vi "LabViewV1.0.0.vi"() -> ()   [LabVIEW 2020]
uses:
  <vilib>/DAQmx/read.llb/DAQmx Read (Analog 2D DBL NChan NSamp).vi
  <vilib>/Analysis/baseanly.llb/Mean (DBL).vi
  <vilib>/DAQmx/miscellaneous.llb/DAQmx Fill In Error Info.vi
  <vilib>/Analysis/NI_AALBase.lvlib
  <resource>/objmgr/daqmx.rc
panel:
  out "Numeric 2":i32
  out "Numeric":i32
  out "index of Module 3":i32
  out "index of Module 2":i32
  out "double precision float":dbl
  out "Time Stamp":timestamp=timestamp(-21600 s since 1904-01-01)
  out "subarray 2":string[](array[string])
  out "index of Module 1":i32
  out "subarray":string[](array[string])
  in  "Counter":dbl
  out ".not. (x .or. y)?":bool
  out "index of element":i32
  out "element":dbl
  out "?":timestamp
  out "Channels":refnum<k21>[](array[refnum])
  out "size(s)":i32
  out "NumDevices":u32
  out "x/y":dbl
  in  "?":T1(tab)
  out "Sampling Status":bool
  in  "Sampling Time":u32=5
  in  "Read Time (s)":u32=60
  in  "Channel List":string(combo)="Temperature"
  out "Read Count Daily":string="0" caption="Timestamp"
  out "Countdown to Read":string="0\n 6:17:48 PM" caption="Timestamp"
  out "?":string="Timestamp"
  out "?":string="File Location"
  out "Timestamp":string="7/26/2020\n 6:17:48 PM"
  in  "Start":bool
  in  "Next Button":bool
  in  "Stop Button 2":bool
  out "Graph Running":bool
  in  "Resolution":u8=10 min=10
  in  "Stop Button":bool
  in  "Play Button":bool
  out "Module 3":bool
  out "Module 2":bool
  out "Module 1":bool
  out "3":bool
  out "2":bool
  out "1":bool
  in  "Running Module":u8=1 min=1 max=3
  in  "Module 3 Task":refnum<k21>="MyTemperatureTask_2"
  out "?":waveform(dbl)(graph)
  in  "Module 3 File Data Location":path=path "E:/KMUTT/Master Degree/labviewjgsee/log/Module3"
  in  "Module 2 File Data Location":path=path "E:/KMUTT/Master Degree/labviewjgsee/log/Module2"
  in  "Module 2 Task":refnum<k21>="MyTemperatureTask_1"
  in  "Module 1 File Data Location":path=path "E:/KMUTT/Master Degree/labviewjgsee/log/Module1"
  in  "Module 1 Task":refnum<k21>="MyTemperatureTask"
  in  "DAQmx Device Name":tag="JGSEE"
  out "Table Module 1":string[][](table)
  out "Table Module 2":string[][](table)
  out "Table Module 3":string[][](table)
  in  "Select Channel Module 1":string(combo)
  out "?":string="Date"
  out "Timestamp 2":string="7/26/2020\n 6:17:48 PM" caption="Timestamp"
  out "Graph Module 1":cluster{timestamp[], dbl[]}[](graph)
  in  "Select Channel Module 2":string(combo)
  out "?":string="Date"
  out "Timestamp 3":string="7/26/2020\n 6:17:48 PM" caption="Timestamp"
  out "Graph Module 2":cluster{timestamp[], dbl[]}[](graph)
  in  "Select Channel Module 3":string(combo)
  out "?":string="Date"
  out "Timestamp 4":string="7/26/2020\n 6:17:48 PM" caption="Timestamp"
  out "Graph Module 3":cluster{timestamp[], dbl[]}[](graph)
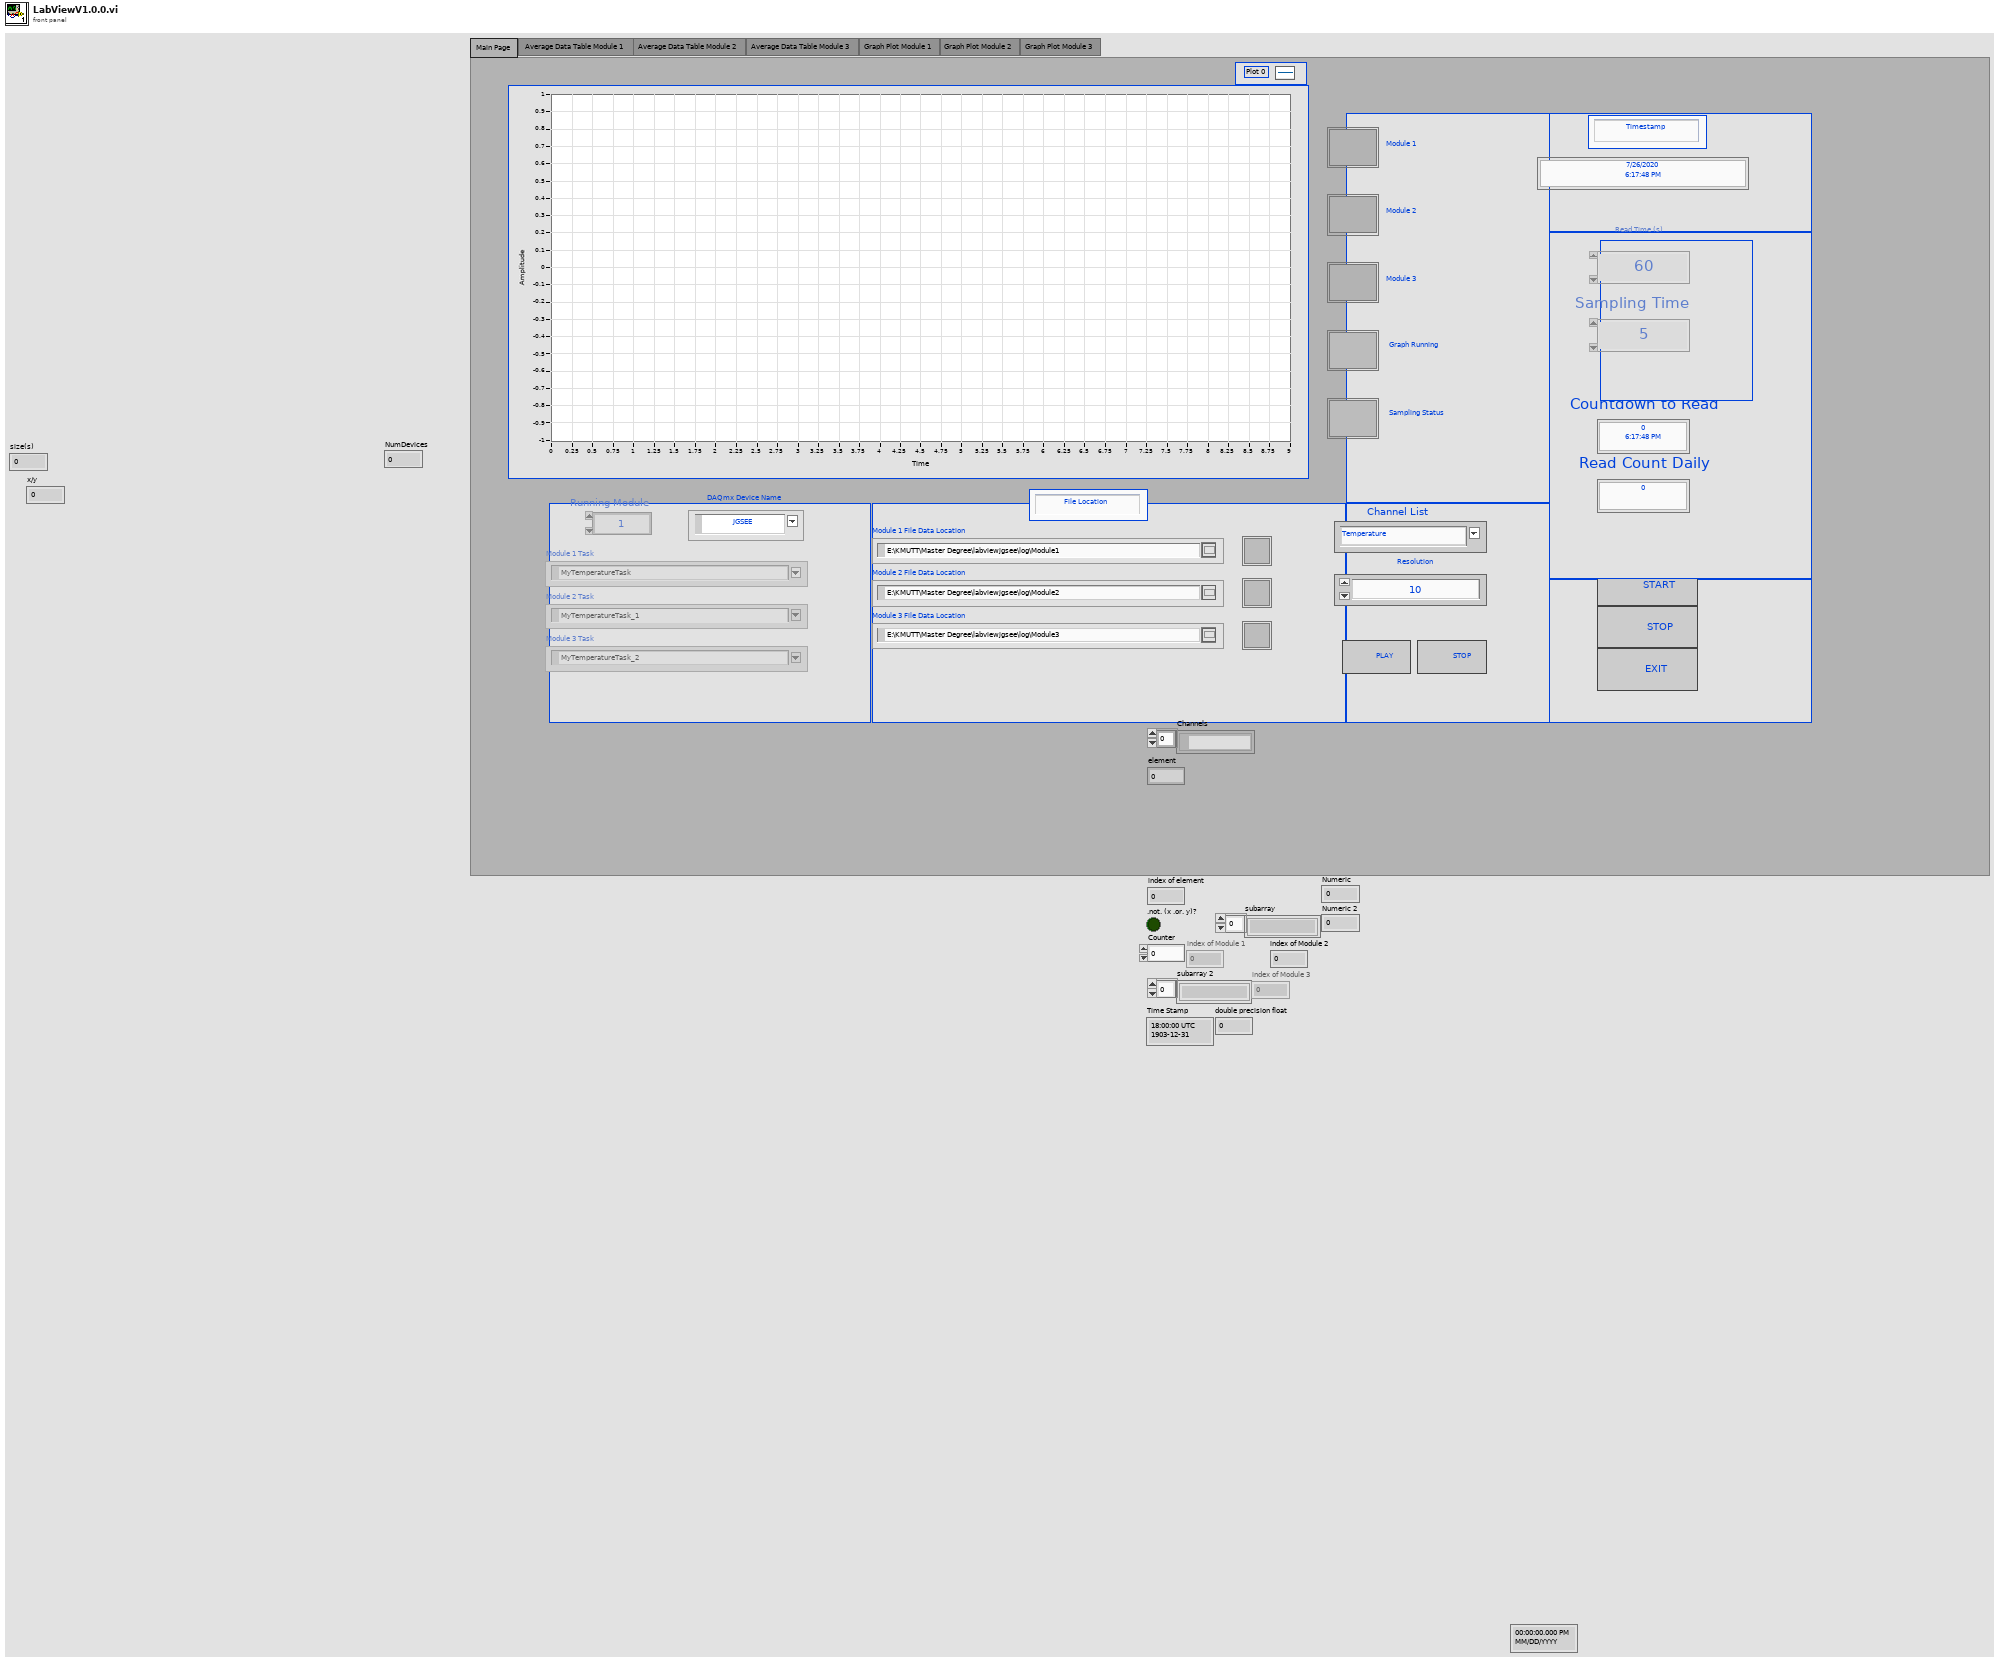
[diagram p1: front panel]
types:
  T1 = enum32{"Main Page ", " Average Data Table Module 1", "Average Data Table Module 2", "Average Data Table Module 3", "Graph Plot Module 1", "Graph Plot Module 2", "Graph Plot Module 3"}
  T2 = enum16{"open", "replace", "create", "open or create", "replace or create", "replace or create with confirmation"}
  T3 = enum8{"Enabled", "Disabled", "Disabled and Grayed Out"}
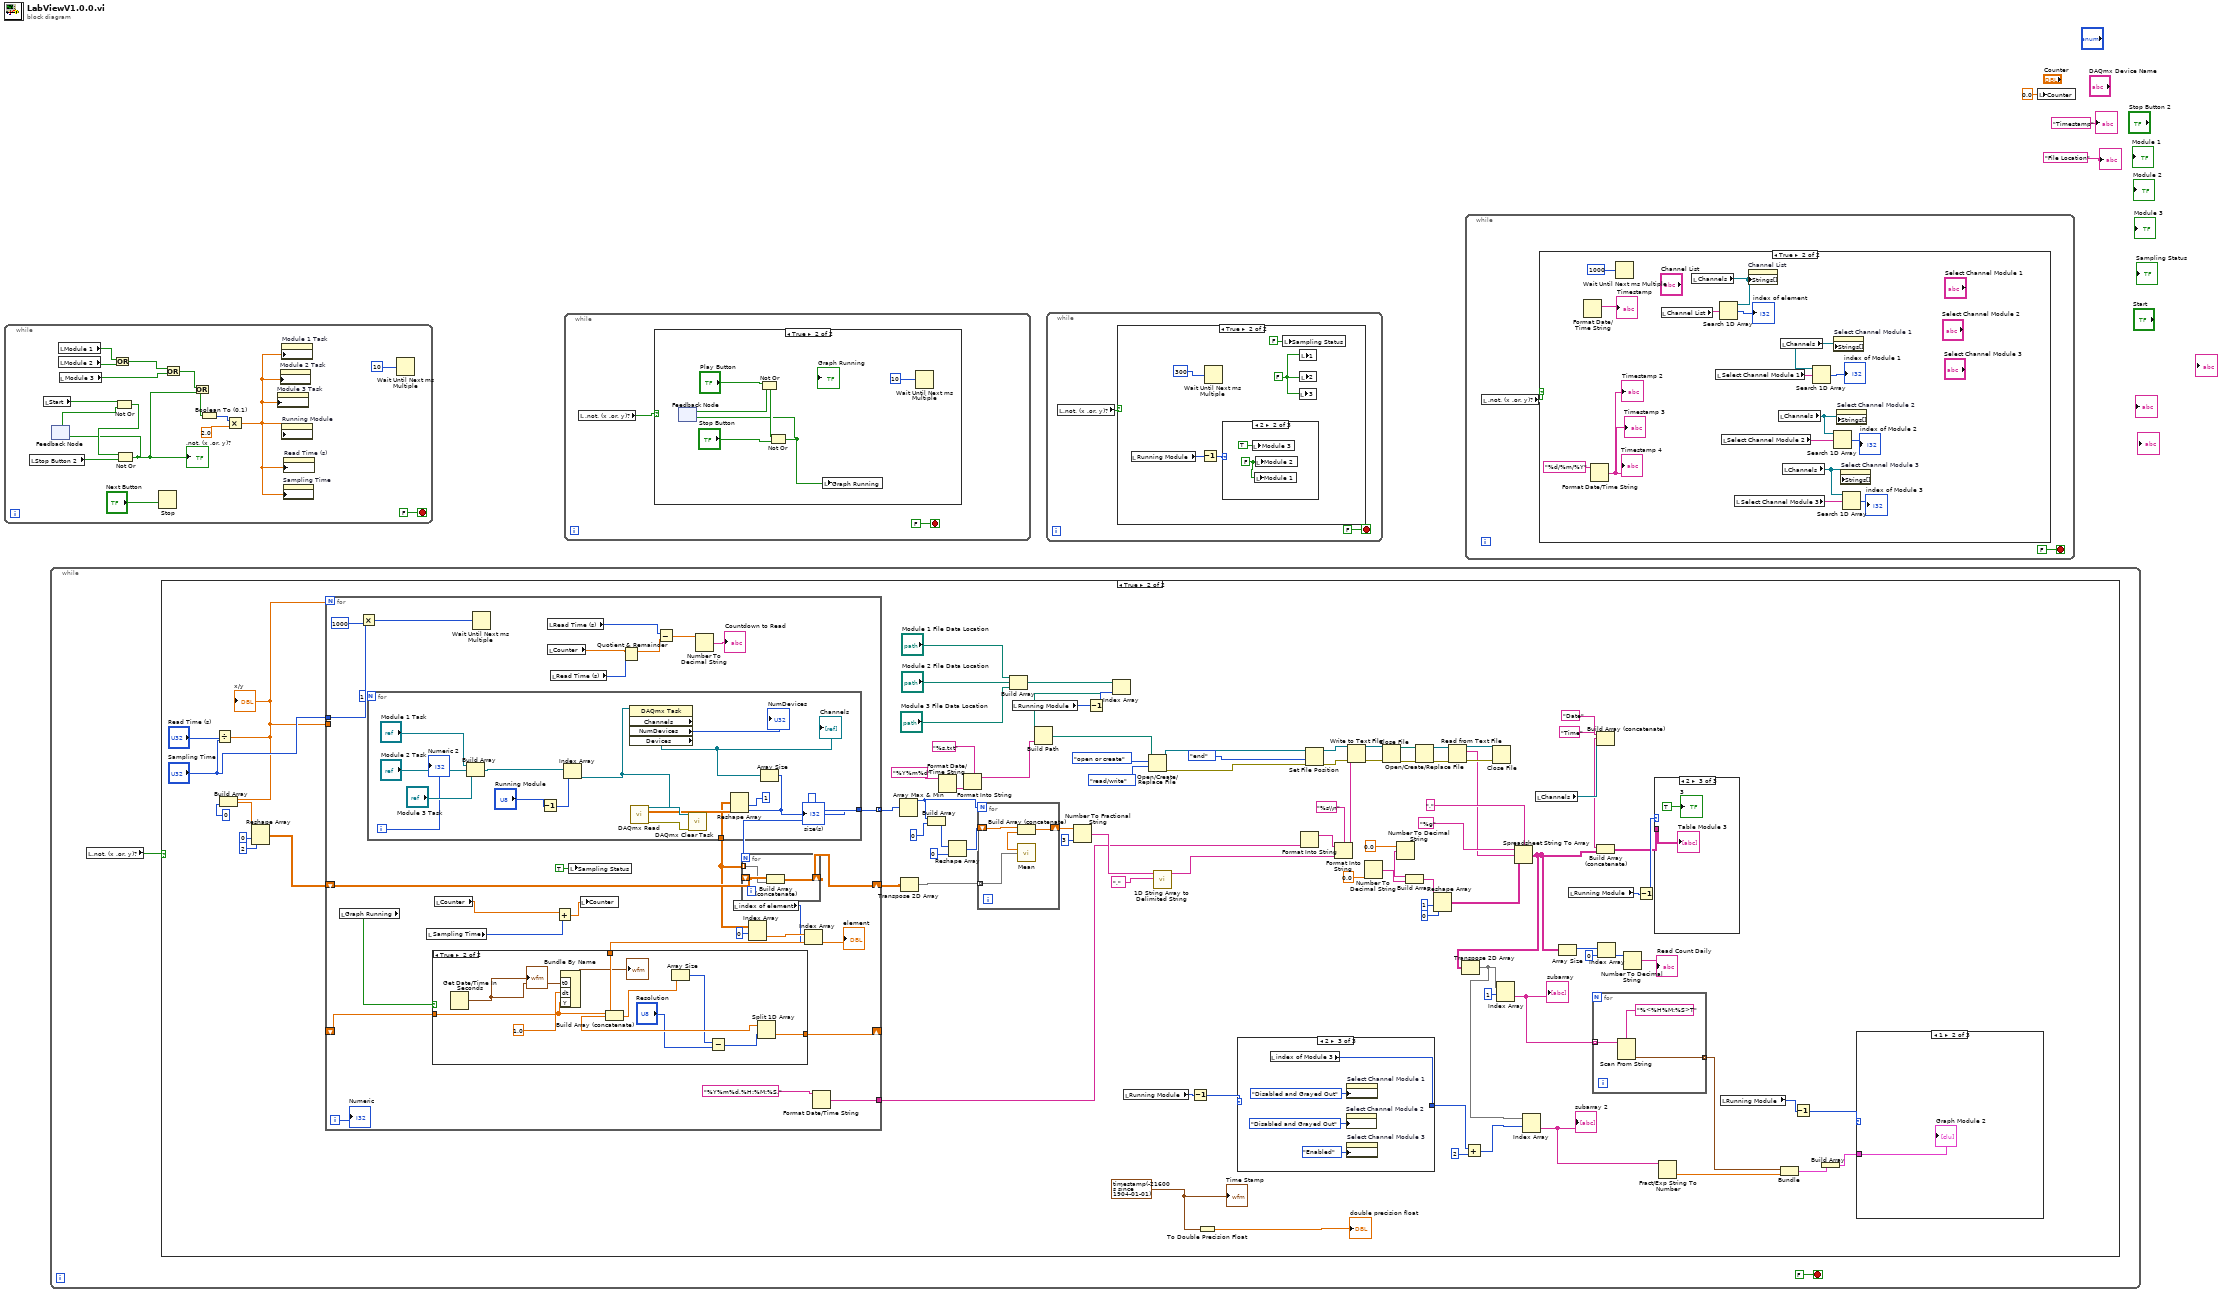
[diagram p0: block diagram]
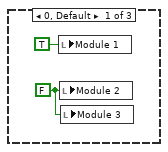
[diagram p4: hidden frame]
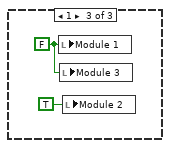
[diagram p5: hidden frame]
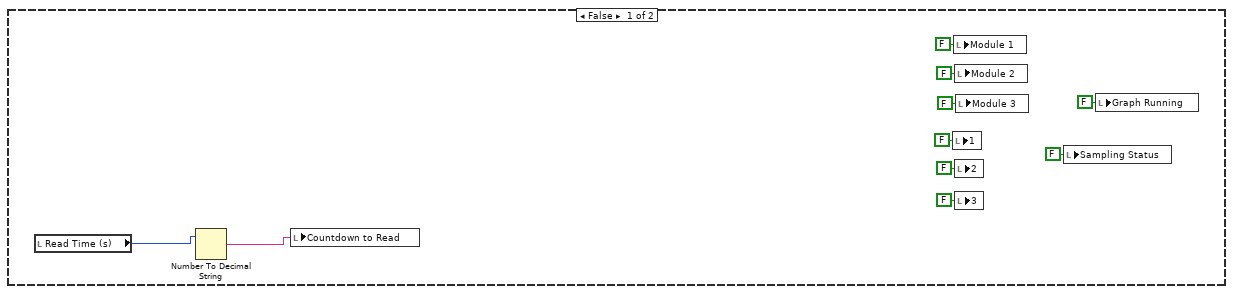
[diagram p7: hidden frame]
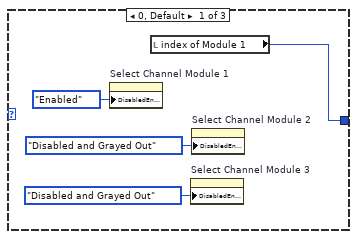
[diagram p8: hidden frame]
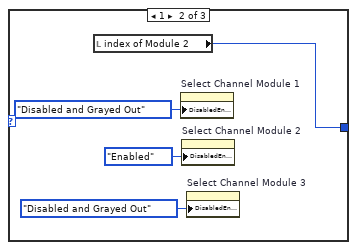
[diagram p9: hidden frame]
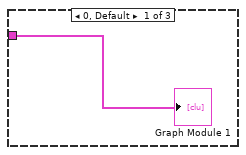
[diagram p10: hidden frame]
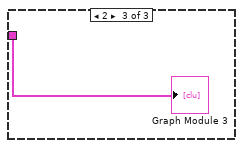
[diagram p11: hidden frame]
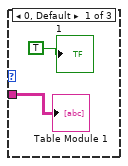
[diagram p12: hidden frame]
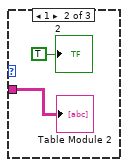
[diagram p13: hidden frame]
diagram:
  n1 = while {
    stop <- FALSE stop-if-true
    n2 = local read "Stop Button 2"() -> (w19:bool)
    n3 = local read "Start"() -> (w15:bool)
    n4 = feedback #1() -> (w17:bool)  [unwired: 1 in]
    n5 = local read "Module 1"() -> (w13:bool)
    n6 = local read "Module 2"() -> (w12:bool)
    n7 = local read "Module 3"() -> (w10:bool)
    n8 = Or(x=w13, y=w12) -> (x .or. y?=w11:bool)
    n9 = Not Or(1:w17, 2:w15) -> (0:w18:bool)
    n10 = Not Or(1:w19, 2:w18) -> (0:w7:bool)
    ".not. (x .or. y)?" <- w7
    n11 = feedback-in #1(w7) -> ()
    n12 = Stop(stop? (T)="Next Button") -> ()
    n13 = Or(x=w11, y=w10) -> (x .or. y?=w9:bool)
    n14 = Or(x=w9, y=w7) -> (x .or. y?=w6:bool)
    n15 = Boolean To (0,1)(Boolean=w6) -> (0, 1=w8:i16)
    n16 = Multiply(x=w8, y=2.0) -> (x*y=w5:dbl)
    n17 = property on="Module 3 Task" class="DAQmxName (strict)"("DisabledEnum"=w5) -> ()  [unwired: 2 in, 2 out]
    n18 = property on="Module 2 Task" class="DAQmxName (strict)"("DisabledEnum"=w5) -> ()  [unwired: 2 in, 2 out]
    n19 = property on="Module 1 Task" class="DAQmxName (strict)"("DisabledEnum"=w5) -> ()  [unwired: 2 in, 2 out]
    n20 = property on="Running Module" class="DigNum (strict)"("DisabledEnum"=w5) -> ()  [unwired: 2 in, 2 out]
    n21 = property on="Sampling Time" class="DigNum (strict)"("DisabledEnum"=w5) -> ()  [unwired: 2 in, 2 out]
    n22 = property on="Read Time (s)" class="DigNum (strict)"("DisabledEnum"=w5) -> ()  [unwired: 2 in, 2 out]
    n23 = Wait Until Next ms Multiple(millisecond multiple=u32 10 ("milliseconds to wait")) -> ()  [unwired: 1 out]
  }
  n24 = while {
    stop <- FALSE stop-if-true
    n25 = local read ".not. (x .or. y)?"() -> (w21:bool)
    n26 = case shown="True" w21 {
      frame False {
        n27 = local read "Read Time (s)"() -> (w24:u32)
        n28 = Number To Decimal String(number=w24) -> (decimal integer string=w23:string)  [unwired: 1 in]
        n29 = local write "Countdown to Read"(w23) -> ()
        n30 = local write "1"(FALSE ("1")) -> ()
        n31 = local write "Module 1"(FALSE ("Module 1")) -> ()
        n32 = local write "Module 2"(FALSE ("Module 2")) -> ()
        n33 = local write "2"(FALSE ("2")) -> ()
        n34 = local write "3"(FALSE ("3")) -> ()
        n35 = local write "Module 3"(FALSE ("Module 3")) -> ()
        n36 = local write "Sampling Status"(FALSE ("Sampling Status")) -> ()
        n37 = local write "Graph Running"(FALSE ("Graph Running")) -> ()
      }
      frame True {
        w42 = timestamp(-21600 s since 1904-01-01)
        n38 = Divide(x="Read Time (s)", y="Sampling Time") -> (x/y=w34:dbl)
        "x/y" <- w34
        n39 = Build Array(w34, 0 ("element")) -> (w107:dbl[])
        n40 = Reshape Array(w107, 0 ("dimension size"), 2 ("dimension size")) -> (w104:dbl[][])
        n41 = for {
          N: w34 -> [_]
          shift-right: [w176] -> w73
          shift-left: w104 -> [w175]
          tunnel: "Sampling Time" -> [w174]
          tunnel: [w172] -> w103 mode=indexing
          shift-right: [w167] -> _
          shift-left: _ -> [w166]
          tunnel: w34 -> [_]
          tunnel: [w153] -> w33
          i -> [w151]
          n42 = local read "Graph Running"() -> (w165:bool)
          n43 = Multiply(x=w174, y=u32 1000) -> (x*y=w149:u32)
          n44 = for {
            N: 1 -> [_]
            tunnel: [w189] -> w172
            tunnel: [w178] -> w171
            i -> [w177]
            n45 = Build Array("Module 1 Task", "Module 2 Task", "Module 3 Task") -> (w184:refnum<k21>[])
            n46 = Decrement(x="Running Module") -> (x-1=w180:u8)
            n47 = Index Array(array=w184, index=w180) -> (element=w183:refnum<k21>)
            n48 = property class="DAQmx Task" props=["Channels", "NumDevices", "Devices"](reference=w183) -> ("Channels"=w179:refnum<k21>[], "NumDevices"=→"NumDevices":u32)  [unwired: 1 in, 3 out]
            "Channels" <- w179
            n49 = call-poly <vilib>:"DAQmx Read.vi"("task/channels in"=w183) -> ("task out"=w191:refnum<k21>, "data"=w188:dbl[][], "error out"=w192:errorcluster)  [unwired: 12 in]
            n50 = call <vilib>:"DAQmx Clear Task.vi"("task in"=w191, "error in"=w192) -> ()  [unwired: 13 in, 1 out]
            n51 = Array Size(array=w179) -> (size(s)=w189:i32)
            "size(s)" <- w189
            n52 = Reshape Array(w188, 1 ("dimension size"), w189) -> (w178:dbl[][])
            "Numeric 2" <- w177
          }
          n53 = local read "Sampling Time"() -> (w161:u32)
          n54 = local read "Counter"() -> (w160:dbl)
          n55 = Wait Until Next ms Multiple(millisecond multiple=w149) -> ()  [unwired: 1 out]
          n56 = local read "Read Time (s)"() -> (w157:u32)
          n57 = local read "Counter"() -> (w154:dbl)
          n58 = local read "Read Time (s)"() -> (w159:u32)
          n59 = Add(x=w160, y=w161) -> (x+y=w162:dbl)
          n60 = local write "Sampling Status"(TRUE ("Sampling Status")) -> ()
          n61 = local write "Counter"(w162) -> ()
          n62 = Quotient & Remainder(x=w154, y=w159) -> (x-y*floor(x/y)=w158:dbl)  [unwired: 1 out]
          n63 = Subtract(x=w157, y=w158) -> (x-y=w156:dbl)
          n64 = Number To Decimal String(number=w156) -> (decimal integer string=→"Countdown to Read":string)  [unwired: 1 in]
          n65 = local read "index of element"() -> (w164:i32)
          n66 = for {
            N: w172 -> [_]
            shift-right: [w204] -> w176
            shift-left: w175 -> [w205]
            tunnel: w171 -> [w203] mode=indexing
            n67 = Build Array (concatenate)(w205, w203) -> (w204:dbl[][])
          }
          n68 = Index Array(array=w171, index (row)=0) -> (element=w169:dbl[])  [unwired: 1 in]
          n69 = Index Array(array=w169, index=w164) -> (element=w168:dbl)
          "element" <- w168
          n70 = case shown="True" w165 {
            tunnel: w168 -> [_ w200]
            tunnel: [_ w197] -> w167
            tunnel: w166 -> [_ w196]
            frame False {
            }
            frame True {
              n71 = Get Date/Time In Seconds() -> (seconds since 1Jan1904=w202:timestamp)
              "?" <- w202
              n72 = Bundle By Name("t0"=w202, "dt"=1.0, "Y"=w196) -> (→"?":waveform(dbl))  [unwired: 1 in]
              n73 = Build Array (concatenate)(w196, w200) -> (w198:dbl[])
              n74 = Array Size(array=w198) -> (size(s)=w194:i32)
              n75 = Subtract(x=w194, y="Resolution") -> (x-y=w195:i32)
              n76 = Split 1D Array(array=w198, index=w195) -> (second subarray=w197:dbl[])  [unwired: 1 out]
            }
          }
          n77 = Format Date/Time String(time format string (%c)="%Y%m%d,%H:%M:%S,") -> (date/time string=w153:string)  [unwired: 2 in]
          "Numeric" <- w151
        }
        n78 = Array Max & Min(array=w103) -> (max value=w100:i32)  [unwired: 3 out]
        n79 = Transpose 2D Array(2D array=w73) -> (transposed array=w102:dbl[][])
        n80 = Build Array(w100, 0 ("element")) -> (w98:i32[])
        n81 = Format Date/Time String(time format string (%c)="%Y%m%d") -> (date/time string=w117:string)  [unwired: 2 in]
        n82 = Reshape Array(w98, 0 ("dimension size")) -> (w97:i32[])
        n83 = Format Into String(format string="%s.txt", w117) -> (resulting string=w115:string)  [unwired: 2 in, 1 out]
        n84 = for {
          N: w100 -> [_]
          tunnel: w102 -> [w209] mode=indexing
          shift-right: [w207] -> w109
          shift-left: w97 -> [w206]
          n85 = call-poly <vilib>:"Mean.vi"("X"=w209) -> ("mean"=w208:dbl)  [unwired: 1 out]
          n86 = Build Array (concatenate)(w206, w208) -> (w207:dbl[])
        }
        n87 = Build Array("Module 1 File Data Location", "Module 2 File Data Location", "Module 3 File Data Location") -> (w66:path[])
        n88 = local read "Running Module"() -> (w67:u8)
        n89 = Number To Fractional String(number=w109, precision (6)=i16 3) -> (F-format string=w110:string[])  [unwired: 2 in]
        n90 = Decrement(x=w67) -> (x-1=w65:u8)
        n91 = Index Array(array=w66, index=w65) -> (element=w64:path)
        n92 = Build Path(base path=w64, name or relative path=w115) -> (appended path=w114:path)
        n93 = local read "Running Module"() -> (w40:u8)
        n94 = Open/Create/Replace File(file path (use dialog)=w114, operation (0:open)=T2."open or create", access (0:read/write)=enum16{"read/write", "read-only", "write-only"}."read/write") -> (refnum out=w95:refnum<file>, error out=w121:errorcluster)  [unwired: 3 in, 1 out]
        n95 = call <vilib>:"1D String Array to Delimited String.vi"("delimiter"="," ("format string"), "string array"=w110) -> ("delimited string"=w113:string)  [unwired: 9 in]
        n96 = Decrement(x=w40) -> (x-1=w39:u8)
        n97 = To Double Precision Float(number=w42) -> (double precision float=→"double precision float":dbl)
        n98 = case shown="2" w39 {
          tunnel: [w128 w132 w136] -> w35
          frame 0, Default {
            n99 = property on="Select Channel Module 1" class="CmbBox"("DisabledEnum"=T3."Enabled" ("Disabled")) -> ()  [unwired: 2 in, 2 out]
            n100 = local read "index of Module 1"() -> (w128:i32)
            n101 = property on="Select Channel Module 3" class="CmbBox"("DisabledEnum"=T3."Disabled and Grayed Out" ("Disabled")) -> ()  [unwired: 2 in, 2 out]
            n102 = property on="Select Channel Module 2" class="CmbBox"("DisabledEnum"=T3."Disabled and Grayed Out" ("Disabled")) -> ()  [unwired: 2 in, 2 out]
          }
          frame 1 {
            n103 = local read "index of Module 2"() -> (w132:i32)
            n104 = property on="Select Channel Module 1" class="CmbBox"("DisabledEnum"=T3."Disabled and Grayed Out" ("Disabled")) -> ()  [unwired: 2 in, 2 out]
            n105 = property on="Select Channel Module 2" class="CmbBox"("DisabledEnum"=T3."Enabled" ("Disabled")) -> ()  [unwired: 2 in, 2 out]
            n106 = property on="Select Channel Module 3" class="CmbBox"("DisabledEnum"=T3."Disabled and Grayed Out" ("Disabled")) -> ()  [unwired: 2 in, 2 out]
          }
          frame 2 {
            n107 = local read "index of Module 3"() -> (w136:i32)
            n108 = property on="Select Channel Module 2" class="CmbBox"("DisabledEnum"=T3."Disabled and Grayed Out" ("Disabled")) -> ()  [unwired: 2 in, 2 out]
            n109 = property on="Select Channel Module 1" class="CmbBox"("DisabledEnum"=T3."Disabled and Grayed Out" ("Disabled")) -> ()  [unwired: 2 in, 2 out]
            n110 = property on="Select Channel Module 3" class="CmbBox"("DisabledEnum"=T3."Enabled" ("Disabled")) -> ()  [unwired: 2 in, 2 out]
          }
        }
        n111 = Format Into String(w33) -> (resulting string=w111:string)  [unwired: 3 in, 1 out]
        n112 = Set File Position(refnum=w95, from (0:start)=enum16{"start", "end", "current"}."end", error in=w121) -> (refnum out=w122:refnum<file>, error out=w120:errorcluster)  [unwired: 1 in]
        n113 = Format Into String(format string="%s\\n", initial string=w111, w113) -> (resulting string=w87:string)  [unwired: 1 in, 1 out]
        n114 = Write to Text File(file (use dialog)=w122, text=w87, error in=w120) -> (refnum out=w94:refnum<file>, error out=w93:errorcluster)  [unwired: 1 in, 1 out]
        n115 = Number To Decimal String(number=0.0 ("element")) -> (decimal integer string=w75:string)  [unwired: 1 in]
        n116 = Close File(refnum=w94, error in=w93) -> (path=w92:path, error out=w91:errorcluster)
        n117 = Number To Decimal String(number=0.0 ("element")) -> (decimal integer string=w77:string)  [unwired: 1 in]
        n118 = Build Array(w77, w75) -> (w79:string[])
        n119 = Open/Create/Replace File(file path (use dialog)=w92, error in=w91) -> (refnum out=w90:refnum<file>, error out=w89:errorcluster)  [unwired: 4 in, 1 out]
        n120 = Reshape Array(w79, 1 ("dimension size"), 0 ("dimension size")) -> (w80:string[][])
        n121 = Read from Text File(file (use dialog)=w90, error in=w89) -> (refnum out=w88:refnum<file>, text=w83:string, error out=w84:errorcluster)  [unwired: 2 in, 1 out]
        n122 = Add(x=w35, y=2) -> (x+y=w48:i32)
        n123 = Close File(refnum=w88, error in=w84) -> ()  [unwired: 2 out]
        n124 = Spreadsheet String To Array(delimiter (Tab)=",", format string="%g", spreadsheet string=w83, array type (2D Dbl)=w80) -> (array=w52:string[][])
        n125 = Transpose 2D Array(2D array=w52) -> (transposed array=w49:string[][])
        n126 = Index Array(array=w49, index (row)=1 ("index")) -> (element=w47:string[])  [unwired: 1 in]
        "subarray" <- w47
        n127 = Index Array(array=w49, index (row)=w48) -> (element=w45:string[])  [unwired: 1 in]
        "subarray 2" <- w45
        n128 = local read "Channels"() -> (w58:refnum<k21>[])
        n129 = Array Size(array=w52) -> (size(s)=w56:i32[])
        n130 = local read "Running Module"() -> (w63:u8)
        n131 = for {
          tunnel: w47 -> [w141] mode=indexing
          tunnel: [w140] -> w43 mode=indexing
          n132 = Scan From String(format string="%<%H%M:%S>T", input string=w141) -> (output 1=w140:timestamp)  [unwired: 3 in, 3 out]
        }
        n133 = Build Array (concatenate)("Date", "Time", w58) -> (w57:string[])
        n134 = Build Array (concatenate)(w57, w52) -> (w61:string[][])
        n135 = Index Array(array=w56, index=0) -> (element=w54:i32)
        n136 = Number To Decimal String(number=w54) -> (decimal integer string=→"Read Count Daily":string)  [unwired: 1 in]
        n137 = Decrement(x=w63) -> (x-1=w62:u8)
        n138 = case shown="2" w62 {
          tunnel: w61 -> [w144 w146 w148]
          frame 0, Default {
            "Table Module 1" <- w144
            "1" <- TRUE ("1")
          }
          frame 1 {
            "Table Module 2" <- w146
            "2" <- TRUE ("2")
          }
          frame 2 {
            "Table Module 3" <- w148
            "3" <- TRUE ("3")
          }
        }
        n139 = Fract/Exp String To Number(string=w45) -> (number=w44:dbl[])  [unwired: 3 in, 1 out]
        n140 = local read "Running Module"() -> (w38:u8)
        n141 = Bundle(w43, w44) -> (w46:cluster{timestamp[], dbl[]})  [unwired: 1 in]
        n142 = Decrement(x=w38) -> (x-1=w37:u8)
        n143 = Build Array(w46) -> (w36:cluster{timestamp[], dbl[]}[])
        n144 = case shown="1" w37 {
          tunnel: w36 -> [w137 w138 w139]
          frame 0, Default {
            "Graph Module 1" <- w137
          }
          frame 1 {
            "Graph Module 2" <- w138
          }
          frame 2 {
            "Graph Module 3" <- w139
          }
        }
        "Time Stamp" <- w42
      }
    }
  }
  n145 = while {
    stop <- FALSE stop-if-true
    n146 = local read ".not. (x .or. y)?"() -> (w210:bool)
    n147 = case shown="True" w210 {
      frame False {
      }
      frame True {
        n148 = feedback #2() -> (w214:bool)  [unwired: 1 in]
        n149 = Not Or(1:w214, 2:"Play Button") -> (0:w215:bool)
        n150 = Not Or(1:"Stop Button", 2:w215) -> (0:w213:bool)
        n151 = feedback-in #2(w213) -> ()
        n152 = local write "Graph Running"(w213) -> ()
        n153 = Wait Until Next ms Multiple(millisecond multiple=u32 10 ("milliseconds to wait")) -> ()  [unwired: 1 out]
      }
    }
  }
  n154 = while {
    stop <- FALSE stop-if-true
    n155 = local read ".not. (x .or. y)?"() -> (w218:bool)
    n156 = case shown="True" w218 {
      frame False {
      }
      frame True {
        w223 = FALSE ("1")
        n157 = local read "Running Module"() -> (w222:u8)
        n158 = Decrement(x=w222) -> (x-1=w221:u8)
        n159 = Wait Until Next ms Multiple(millisecond multiple=u32 300 ("milliseconds to wait")) -> ()  [unwired: 1 out]
        n160 = case shown="2" w221 {
          frame 0, Default {
            w226 = FALSE ("Module 2")
            n161 = local write "Module 1"(TRUE ("Module 1")) -> ()
            n162 = local write "Module 2"(w226) -> ()
            n163 = local write "Module 3"(w226) -> ()
          }
          frame 2 {
            w228 = FALSE ("Module 2")
            n164 = local write "Module 3"(TRUE ("Module 3")) -> ()
            n165 = local write "Module 1"(w228) -> ()
            n166 = local write "Module 2"(w228) -> ()
          }
          frame 1 {
            w230 = FALSE ("Module 1")
            n167 = local write "Module 1"(w230) -> ()
            n168 = local write "Module 3"(w230) -> ()
            n169 = local write "Module 2"(TRUE ("Module 2")) -> ()
          }
        }
        n170 = local write "Sampling Status"(FALSE ("Sampling Status")) -> ()
        n171 = local write "3"(w223) -> ()
        n172 = local write "1"(w223) -> ()
        n173 = local write "2"(w223) -> ()
      }
    }
  }
  n174 = while {
    stop <- FALSE stop-if-true
    n175 = local read ".not. (x .or. y)?"() -> (w231:bool)
    n176 = case shown="True" w231 {
      frame False {
      }
      frame True {
        n177 = Format Date/Time String() -> (date/time string=→"Timestamp":string)  [unwired: 3 in]
        n178 = Format Date/Time String(time format string (%c)="%d/%m/%Y") -> (date/time string=→"Timestamp 2" →"Timestamp 3" →"Timestamp 4":string)  [unwired: 2 in]
        n179 = Wait Until Next ms Multiple(millisecond multiple=u32 1000 ("milliseconds to wait")) -> ()  [unwired: 1 out]
        n180 = local read "Channel List"() -> (w247:string)
        n181 = local read "Channels"() -> (w248:refnum<k21>[])
        n182 = local read "Select Channel Module 1"() -> (w244:string)
        n183 = Search 1D Array(1D array=w248, element=w247) -> (index of element=→"index of element":i32)  [unwired: 1 in]
        n184 = local read "Select Channel Module 2"() -> (w242:string)
        n185 = local read "Select Channel Module 3"() -> (w239:string)
        n186 = property on="Channel List" class="CmbBox"("Strings[]"=w248) -> ()  [unwired: 2 in, 2 out]
        n187 = local read "Channels"() -> (w241:refnum<k21>[])
        n188 = local read "Channels"() -> (w245:refnum<k21>[])
        n189 = local read "Channels"() -> (w238:refnum<k21>[])
        n190 = Search 1D Array(1D array=w245, element=w244) -> (index of element=→"index of Module 1":i32)  [unwired: 1 in]
        n191 = Search 1D Array(1D array=w241, element=w242) -> (index of element=→"index of Module 2":i32)  [unwired: 1 in]
        n192 = property on="Select Channel Module 1" class="CmbBox"("Strings[]"=w245) -> ()  [unwired: 2 in, 2 out]
        n193 = property on="Select Channel Module 2" class="CmbBox"("Strings[]"=w241) -> ()  [unwired: 2 in, 2 out]
        n194 = property on="Select Channel Module 3" class="CmbBox"("Strings[]"=w238) -> ()  [unwired: 2 in, 2 out]
        n195 = Search 1D Array(1D array=w238, element=w239) -> (index of element=→"index of Module 3":i32)  [unwired: 1 in]
      }
    }
  }
  n196 = local write "Counter"(0.0 ("Counter")) -> ()
  "?" <- "File Location" ("String")
  "?" <- "Timestamp"
